vi "Get configuration chain.vi"(8 "error in (no error)":errorcluster, 11 "WaveformBase in":refnum<class "Waveform.lvclass">) -> (0 "error out":errorcluster, 1 "class name":string[](array[string]), 2 "configuration chain":variant[](array[variant]), 3 "WaveformBase out":refnum<class "Waveform.lvclass">)   [LabVIEW 2012, in "Waveform.lvclass"]
doc: "Returns an array of variants containing the configuration clusters of each class in the inheritance chain (lowest child class first), together with an array of all class names in the inheritance chain.\n\nFor classes without configuration cluster, the configuration chain contains empty variants."
uses:
  Waveform.lvclass
  <vilib>/Distrio/Murmex/Murmex/Murmex.lvclass
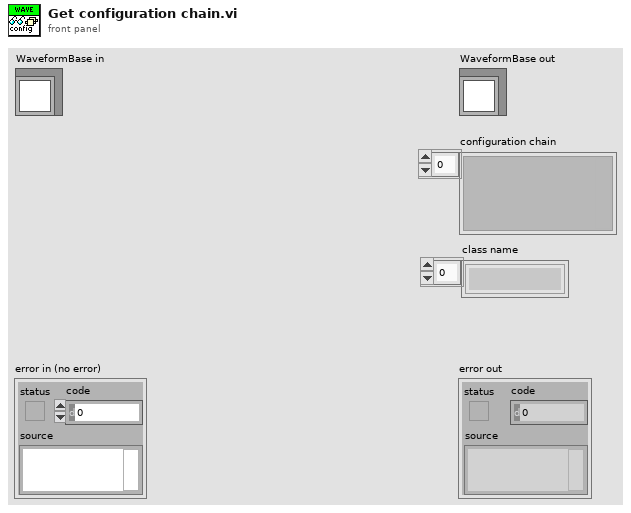
[diagram p1: front panel]
types:
  T1 = typedef "Waveform.lvclass/configuration.ctl" = cluster{"Counter":T2, "analog out":T3, "related components":T4}
  T2 = typedef "Waveform.lvclass/counter_config.ctl" = cluster{"Counter 1":cluster{"Duty cycle":dbl, "Frequency":dbl, "Counter":tag, "Output Terminal":tag}, "Counter 2":cluster{"Duty cycle":dbl, "Frequency":dbl, "Counter":tag, "Output Terminal":tag}}
  T3 = typedef "Waveform.lvclass/AO_config.ctl" = cluster{"AO0":cluster{"min Voltage":dbl, "max Voltage":dbl, "Physical Channel":tag, "trigger edge":i32, "trigger source":tag}, "AO1":cluster{"min Voltage":dbl, "max Voltage":dbl, "Physical Channel":tag, "trigger edge":i32, "trigger source":tag}, "AO2":cluster{"min Voltage":dbl, "max Voltage":dbl, "Physical Channel":tag, "trigger edge":i32, "trigger source":tag}}
  T4 = typedef "Waveform.lvclass/related components.ctl" = cluster{"Camera 1":string, "Camera 2":string, "Camera 3":string}
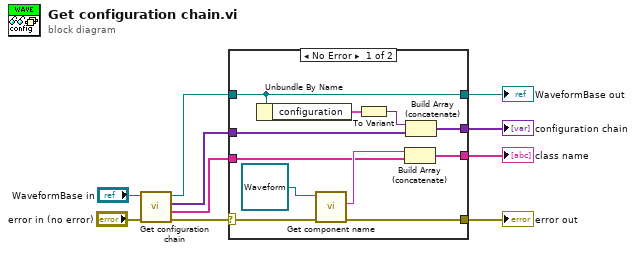
[diagram p0: block diagram]
diagram:
  n1 = call-parent "Get configuration chain.vi"("error in (no error)"="error in (no error)", "MurmexBase in"="WaveformBase in") -> ("error out"=w8:errorcluster, "class name"=w2:string[], "configuration chain"=w1:variant[], "MurmexBase out"=w6:refnum<class "Waveform.lvclass">)  [unwired: 6 in]
  n2 = case shown="No Error" w8 {
    selector: w8 -> [w20 w24]
    tunnel: [w19 w24] -> w7
    tunnel: w6 -> [w16 w25]
    tunnel: [w16 w25] -> w5
    tunnel: [w15 w22] -> w4
    tunnel: [w14 w23] -> w3
    tunnel: w2 -> [w12 w23]
    tunnel: w1 -> [w11 w22]
    frame No Error {
      n3 = Unbundle By Name(w16) -> ("configuration"=w17:T1)
      n4 = call <vilib>:"Get component name.vi"("error in (no error)"=w20, "Murmex in"=refnum<class "Waveform.lvclass"> refnum ("Waveform")) -> ("error out"=w19:errorcluster, "component name"=w13:string)  [unwired: 7 in, 1 out]
      n5 = To Variant(anything=w17) -> (Variant=w18:variant)
      n6 = Build Array (concatenate)(w13, w12) -> (w14:string[])
      n7 = Build Array (concatenate)(w18, w11) -> (w15:variant[])
    }
    frame Error {
    }
  }
  "error out" <- w7
  "WaveformBase out" <- w5
  "configuration chain" <- w4
  "class name" <- w3
